vi "Init Nodes.vi"(8 "error in (no error)":errorcluster, 11 "Debug GUI Module in":refnum<class "Debug GUI Module.lvclass">) -> (0 "error out":errorcluster, 3 "Debug GUI Module out":refnum<class "Debug GUI Module.lvclass">)   [LabVIEW 2020, in "VolatusGUI.lvlib" / "Debug GUI Module.lvclass"]
uses:
  Debug GUI Module.lvclass
  C:/dev/lv20CE/relink/lv-volatus/Volatus/Module/Module.lvclass
  VolatusConfig/Meta Type.ctl
  Debug GUI Module.lvclass/Debug GUI Module.ctl
  Volatus/Module/Module.lvclass/Module.ctl
  Volatus/VolatusAPI/VolatusAPI.lvclass/VolatusAPI.ctl
  VolatusConfig/VolatusConfigElement/VolatusConfigElement.lvclass/VolatusConfigElement.ctl
  Node Status.ctl
  Volatus/Module Status.ctl
  Volatus/Module/State.ctl
  VolatusConfig/VolatusConfigElement/Element.vi
  VolatusConfig/Node/Node Config.lvclass
  C:/dev/lv20CE/relink/lv-volatus/VolatusConfig/VolatusConfigElement/VolatusConfigElement.lvclass
  lv-cdm/CDM-Config/Config Lookup/Match Meta.vi
  lv-cdm/CDM-Config/Config Element/Owner.vi
  lv-cdm/CDM-Config/Config Manager/Lookup Descendant.vi
  lv-cdm/CDM-Config/Config Filter/Config Lookup.lvclass
  VolatusConfig/VolatusConfigElement/VolatusConfigElement.lvclass
  VolatusConfig/VolatusConfig.lvlib
  lv-cdm/CDM-Config/Config Element/Config Element.lvclass
  Volatus/Module/Module.lvclass
  Volatus/Volatus.lvlib
  Volatus/VolatusAPI/VolatusAPI.lvclass
  C:/dev/lv20CE/relink/lv-volatus/VolatusGUI/Debug GUI Module/Debug GUI Module.lvclass
  C:/dev/lv20CE/relink/lv-volatus/VolatusConfig/Node/Node Config.lvclass
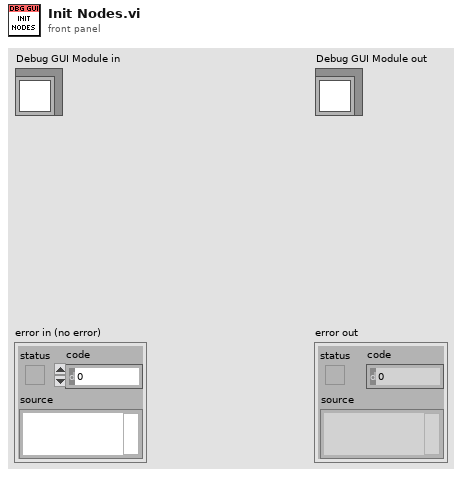
[diagram p1: front panel]
types:
  T1 = typedef "VolatusConfig.lvlib/Meta Type.ctl" = enum16{"UNKNOWN", "VL_System", "VL_Cluster", "VL_Node", "VL_Task", "VL_Group", "VL_Channel", "VL_Task_List", "VL_Scaling", "VL_Sensor", "VL_Sensor_List", "VL_Scale"}
  T2 = typedef "VolatusGUI.lvlib/Debug GUI Module.lvclass/Node Status.ctl" = cluster{"URL":string, "Status Tree":map{string[], T3}}
  T3 = typedef "Volatus.lvlib/Module Status.ctl" = cluster{"Hierarchy":string[], "State":T4, "Substatus":map{string, string}, "Metrics":map{string, dbl}}
  T4 = typedef "Volatus.lvlib/Module.lvclass/State.ctl" = enum16{"Unknown", "Launched", "Starting", "Running", "Stopping", "Stopped", "Error - Starting", "Error - Run", "Error - Stopping"}
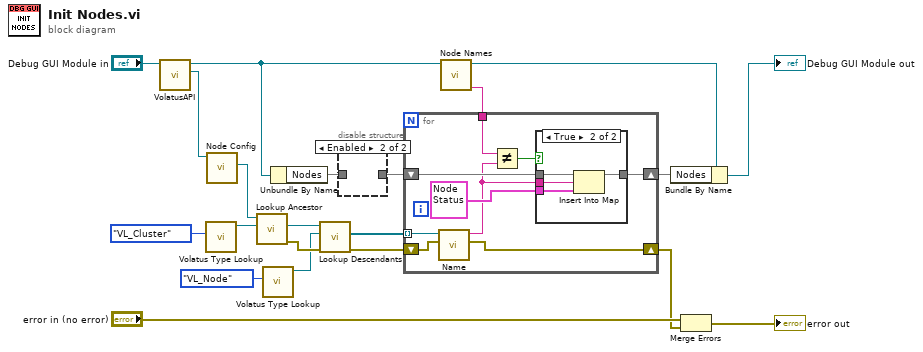
[diagram p0: block diagram]
diagram:
  n1 = call "VolatusAPI.vi"("Module in"="Debug GUI Module in") -> ("VolatusAPI"=w3:refnum<class "VolatusAPI.lvclass">, "Module out"=w5:refnum<class "Debug GUI Module.lvclass">)  [unwired: 9 in]
  n2 = call "Volatus Type Lookup.vi"("Meta Type"=Meta_Type."VL_Cluster") -> ("Config Lookup out"=w19:refnum<class "Config Lookup.lvclass">)  [unwired: 9 in, 1 out]
  n3 = call "Node Config.vi"("VolatusAPI in"=w3) -> ("Node Config"=w4:refnum<class "Node Config.lvclass">)  [unwired: 9 in, 1 out]
  n4 = call "Lookup Ancestor.vi"("Lookup"=w19, "VolatusConfigElement in"=w4) -> ("error out"=w21:errorcluster, "Ancestor"=w16:refnum<class "Config Element.lvclass">)  [unwired: 7 in, 1 out]
  n5 = call "Volatus Type Lookup.vi"("Meta Type"=Meta_Type."VL_Node") -> ("Config Lookup out"=w9:refnum<class "Config Lookup.lvclass">)  [unwired: 9 in, 1 out]
  n6 = Unbundle By Name(w5) -> ("Nodes"=w11:map{string, T2})
  n7 = call "Lookup Descendants.vi"("error in (no error)"=w21, "Lookup"=w9, "Config Element in"=w16) -> ("error out"=w14:errorcluster, "Descendants"=w15:refnum<class "Config Element.lvclass">[])  [unwired: 6 in, 1 out]
  n8 = disable-structure shown="Enabled" {
    disable-tunnel: [w22 _] -> w12
    disable-tunnel: w11 -> [w22 _]
    frame Disabled {
    }
    frame Enabled {
    }
  }
  n9 = call "Node Names.vi"("Module in"=w5) -> ("Node"=w1:string, "Module out"=w2:refnum<class "Debug GUI Module.lvclass">)  [unwired: 6 in, 3 out]
  n10 = for {
    tunnel: w15 -> [w31] mode=indexing
    shift-right: [w27] -> w7
    shift-left: w14 -> [w30]
    shift-right: [w28] -> w10
    shift-left: w12 -> [w29]
    tunnel: w1 -> [w24]
    n11 = call "Name.vi"("error in (no error)"=w30, "Config Element in"=w31) -> ("error out"=w27:errorcluster, "Name"=w25:string)  [unwired: 8 in]
    n12 = Not Equal?(x=w24, y=w25) -> (x != y?=w23:bool)
    n13 = case shown="True" w23 {
      tunnel: w29 -> [w32 w36]
      tunnel: [w32 w35] -> w28
      tunnel: T2 {"URL"="", "Status Tree"={}} ("value") -> [_ w34]
      tunnel: w25 -> [_ w33]
      frame False {
      }
      frame True {
        n14 = Insert Into Map(map in=w36, key=w33, value=w34) -> (map out=w35:map{string, T2})  [unwired: 2 out]
      }
    }
  }
  n15 = Bundle By Name(cluster=w2, "Nodes"=w10) -> (→"Debug GUI Module out":refnum<class "Debug GUI Module.lvclass">)
  n16 = Merge Errors("error in (no error)", w7) -> (→"error out":errorcluster)
